vi "Init.vi"(8 "error in (no error)":errorcluster, 11 "reference in":refnum<class "TestView_Tree_Single.lvclass">) -> (0 "error out":errorcluster, 3 "reference in":refnum<class "TestView_Tree_Single.lvclass">)   [LabVIEW 2022 SP3, in "TestView_Tree_Single.lvlib" / "TestView_Tree_Single.lvclass"]
uses:
  TestView_Tree_Single.lvclass
  Components/TestView_Base.lvlibp/ViewStatus.ctl
  Components/TestView_Base.lvlibp/TestView_Base.lvclass
  Components/ViPER.lvlibp/ViPER.lvclass
  C:/Projects/Medulla/ViPER/Examples/Flux_Capacitor_Tester/Components/ViPER.lvlibp/ViPER.lvclass
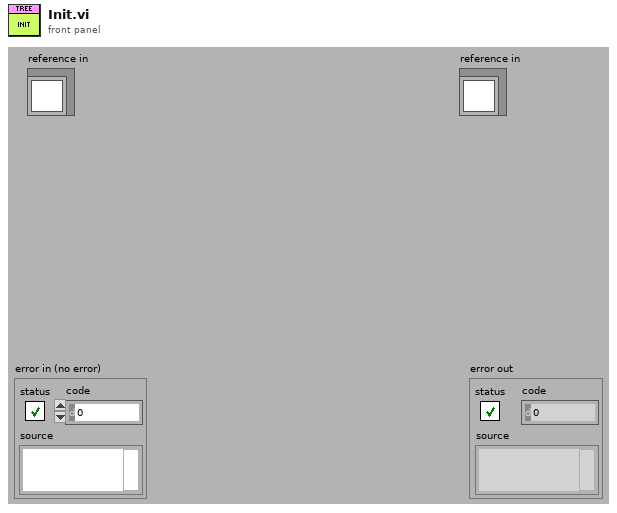
[diagram p1: front panel]
types:
  T1 = typedef "TestView_Base.lvlibp/TestView_Base.lvclass/ViewStatus.ctl" = enum16{"Testing", "Ready", "Logout", "Login", "PASS", "FAIL", "FAULT", "ABORTED"}
  T2 = typedef "TestView_Tree_Single.lvlib/TestView_Tree_Single.lvclass/ObjectAttributes.ctl" = cluster{"Front Panel":refnum<vi>, "Last_Item":string, "Config":T3, "Title":string, "User":string, "TreeRef":refnum<vi>, "Active DUT":i32, "Status":T1, "SN":string, "Spec":string}
  T3 = typedef "TestView_Tree_Single.lvlib/TestView_Tree_Single.lvclass/Config.ctl" = cluster{"default":string}
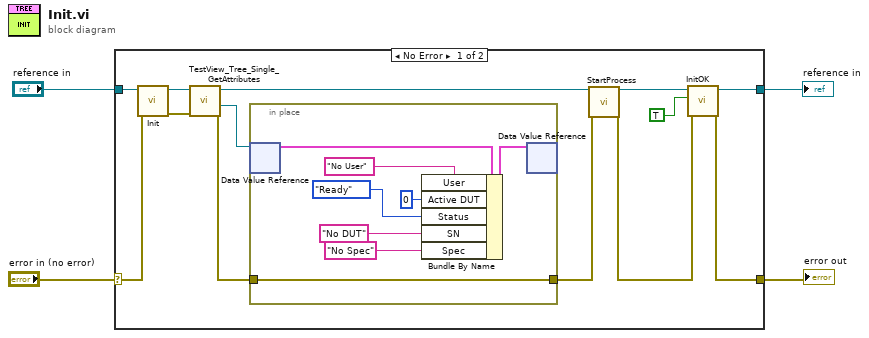
[diagram p0: block diagram]
diagram:
  n1 = case shown="No Error" "error in (no error)" {
    selector: "error in (no error)" -> [w16 w27]
    tunnel: [w12 w27] -> w3
    tunnel: [w14 w26] -> w1
    tunnel: "reference in" -> [w17 w26]
    frame No Error {
      n2 = call-parent "Init.vi"("error in (no error)"=w16, "reference in"=w17) -> ("error out"=w8:errorcluster, "reference in"=w10:refnum<class "TestView_Tree_Single.lvclass">)  [unwired: 8 in]
      n3 = call "TestView_Tree_Single_GetAttributes.vi"("error in (no error)"=w8, "reference in"=w10) -> ("error out"=w6:errorcluster, "DataRef"=w7:refnum<data-value>, "reference out"=w9:refnum<class "TestView_Tree_Single.lvclass">)  [unwired: 6 in, 1 out]
      n4 = in-place {
        in-place-border: w6 -> [w22]
        in-place-border: [w22] -> w5
        n5 = in-place-dvr #1(w7) -> (w24:T2)  [unwired: 1 out]
        n6 = Bundle By Name(cluster=w24, "User"="No User", "Active DUT"=0, "Status"=ViewStatus."Ready", "SN"="No DUT", "Spec"="No Spec" ("SN")) -> (w23:T2)
        n7 = in-place-dvr #1(w23) -> ()  [unwired: 2 out]
      }
      n8 = call "StartProcess.vi"("reference in"=w9, "error in (no error)"=w5) -> ("reference out"=w15:refnum<class "TestView_Tree_Single.lvclass">, "error out"=w13:errorcluster)  [unwired: 16 in]
      n9 = call "InitOK.vi"("error in (no error)"=w13, "Init OK?"=TRUE, "reference in"=w15) -> ("error out"=w12:errorcluster, "reference out"=w14:refnum<class "TestView_Tree_Single.lvclass">)  [unwired: 7 in]
    }
    frame Error {
    }
  }
  "error out" <- w3
  "reference in" <- w1
